vi "XY Graph Get Caption.vi"(2 "XYGraph":refnum<vi>) -> (7 "Graph Caption":string)   [LabVIEW 2019]
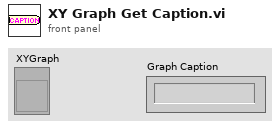
[diagram p1: front panel]
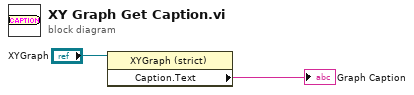
[diagram p0: block diagram]
diagram:
  n1 = property class="XYGraph (strict)"(reference="XYGraph") -> ("Caption.Text"=→"Graph Caption":string)  [unwired: 1 in, 2 out]
